vi "index (2).vi"() -> (1 "XY graph visual":cluster{dbl[], dbl[]}(graph))   [LabVIEW 2026]
uses:
  <userlib>/Status.ctl
  <vilib>/Instr/_visa.llb/VISA Flush IO Buffer Mask.ctl
  <vilib>/Instr/_visa.llb/VISA Configure Serial Port (Instr).vi
  <vilib>/Analysis/3filter.llb/Butterworth Filter (DBL).vi
  <vilib>/measure/maspectr.llb/FFT Spectrum (Mag-Phase) for N Chan.vi
  <vilib>/measure/NI_MAPro.lvlib
  <vilib>/Analysis/NI_AALBase.lvlib
panel:
  out "read buffer":string
  out "CRC Error":bool
  out "Spectrum":cluster{"f0":dbl, "df":dbl, "magnitude":dbl[]}[](graph)
  in  "EditCluster":T1={"Horní mezní frekvence"=0.45000000000000007, "Dolní mezní frekvence"=0.0, "filter type"=enum."Lowpass", "applyFilter"=FALSE, "removeFilter"=FALSE, "undoFIlter"=FALSE} {"Horní mezní frekvence" format="%0.2f"}
  out "Waveform Graph Edit":waveform(dbl)[](graph)
  out "Zobrazeni typu signalu":cluster{string, string}
  in  "Exit Button":bool
  out "NewVal":bool
  in  "MereniAZpracovaniSwitch":bool
  in  "Cluster":T2={"Zařízení"="", "Cesta k uloženému souboru"=path "", "Vzorkovací frekvence"=enum."1000", "Record Button"=FALSE, "Stop Button"=FALSE, "A1 signál"=enum."EMG", "A2 signál"=enum."EMG", "A3 signál"=enum."EMG", "A4 signál"=enum."EMG", "A5 signál"=enum."EMG", "A6 signál"=enum."EMG", "Pin s připojeným signálem"=enum."A1"}
  in  "DO 4":bool
  in  "DO 3":bool
  in  "DO 2":bool
  in  "DO 1":bool
  out "tdms file":refnum<k34>
  out "Ylabel and Plot name":cluster{string, string}
  out "Sample Rate Numeric":i32
  out "Consumer":i32
  out "producer":i32
  in  "error in (no error)":errorcluster
  out "Sync Stop":bool=TRUE
  # "Aplikace pro měření a zpracování dat na platformě PLUX BITalino"
  # "Hz"
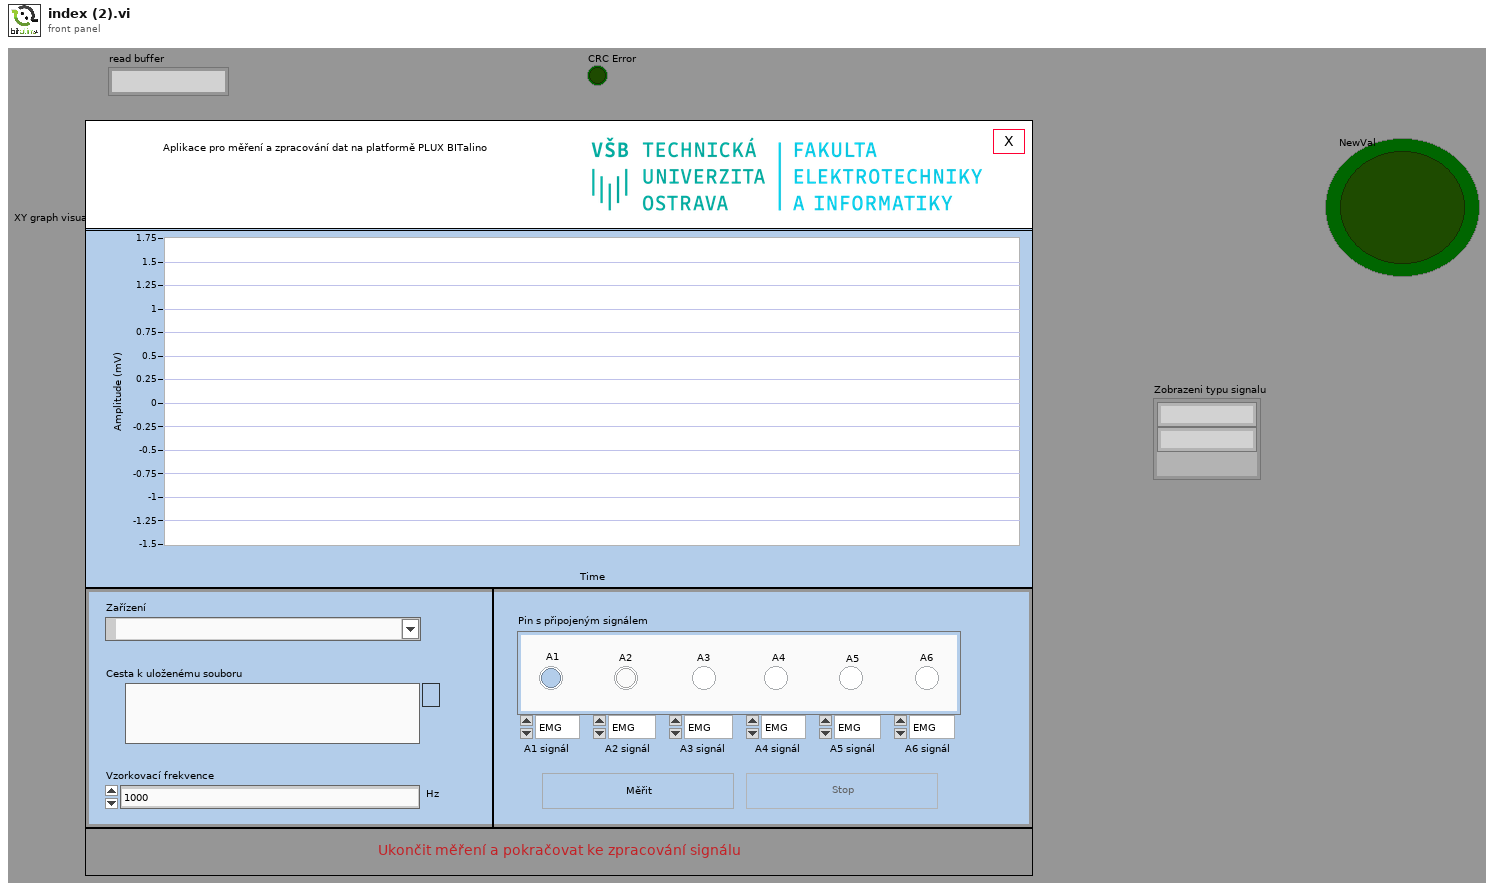
[diagram p1: front panel]
types:
  T1 = cluster{"Horní mezní frekvence":dbl, "Dolní mezní frekvence":dbl, "filter type":enum32{"Lowpass", "Highpass", "Bandpass", "Bandstop"}, "applyFilter":bool, "removeFilter":bool, "undoFIlter":bool}
  T2 = cluster{"Zařízení":refnum<visa-resource-name>, "Cesta k uloženému souboru":path, "Vzorkovací frekvence":enum16{"1", "10", "100", "1000"}, "Record Button":bool, "Stop Button":bool, "A1 signál":enum16{"EMG", "ECG", "EEG", "EDA", "ACC"}, "A2 signál":enum16{"EMG", "ECG", "EEG", "EDA", "ACC"}, "A3 signál":enum16{"EMG", "ECG", "EEG", "EDA", "ACC"}, "A4 signál":enum16{"EMG", "ECG", "EEG", "EDA", "ACC"}, "A5 signál":enum16{"EMG", "ECG", "EEG", "EDA", "ACC"}, "A6 signál":enum16{"EMG", "ECG", "EEG", "EDA", "ACC"}, "Pin s připojeným signálem":enum32{"A1", "A2", "A3", "A4", "A5", "A6"}}
  T3 = enum8{"Enabled", "Disabled", "Disabled and Grayed Out"}
  T4 = enum16{"open", "open or create", "create or replace", "create", "open (read-only)"}
  T5 = typedef "Status.ctl" = enum16{"Initialize", "Edit", "Standby", "Recording", "Exit"}
  T6 = typedef "VISA Flush IO Buffer Mask.ctl" = u16
  T7 = enum32{"Lowpass", "Highpass", "Bandpass", "Bandstop"}
  T8 = cluster{"A1 signál":enum16{"EMG", "ECG", "EEG", "EDA", "ACC"}, "A2 signál":enum16{"EMG", "ECG", "EEG", "EDA", "ACC"}, "A3 signál":enum16{"EMG", "ECG", "EEG", "EDA", "ACC"}, "A4 signál":enum16{"EMG", "ECG", "EEG", "EDA", "ACC"}, "A5 signál":enum16{"EMG", "ECG", "EEG", "EDA", "ACC"}, "A6 signál":enum16{"EMG", "ECG", "EEG", "EDA", "ACC"}}
  T9 = cluster{"Result":dbl, "Result":dbl, "Result":dbl, "Result":dbl, "Result":dbl, "Result":dbl}
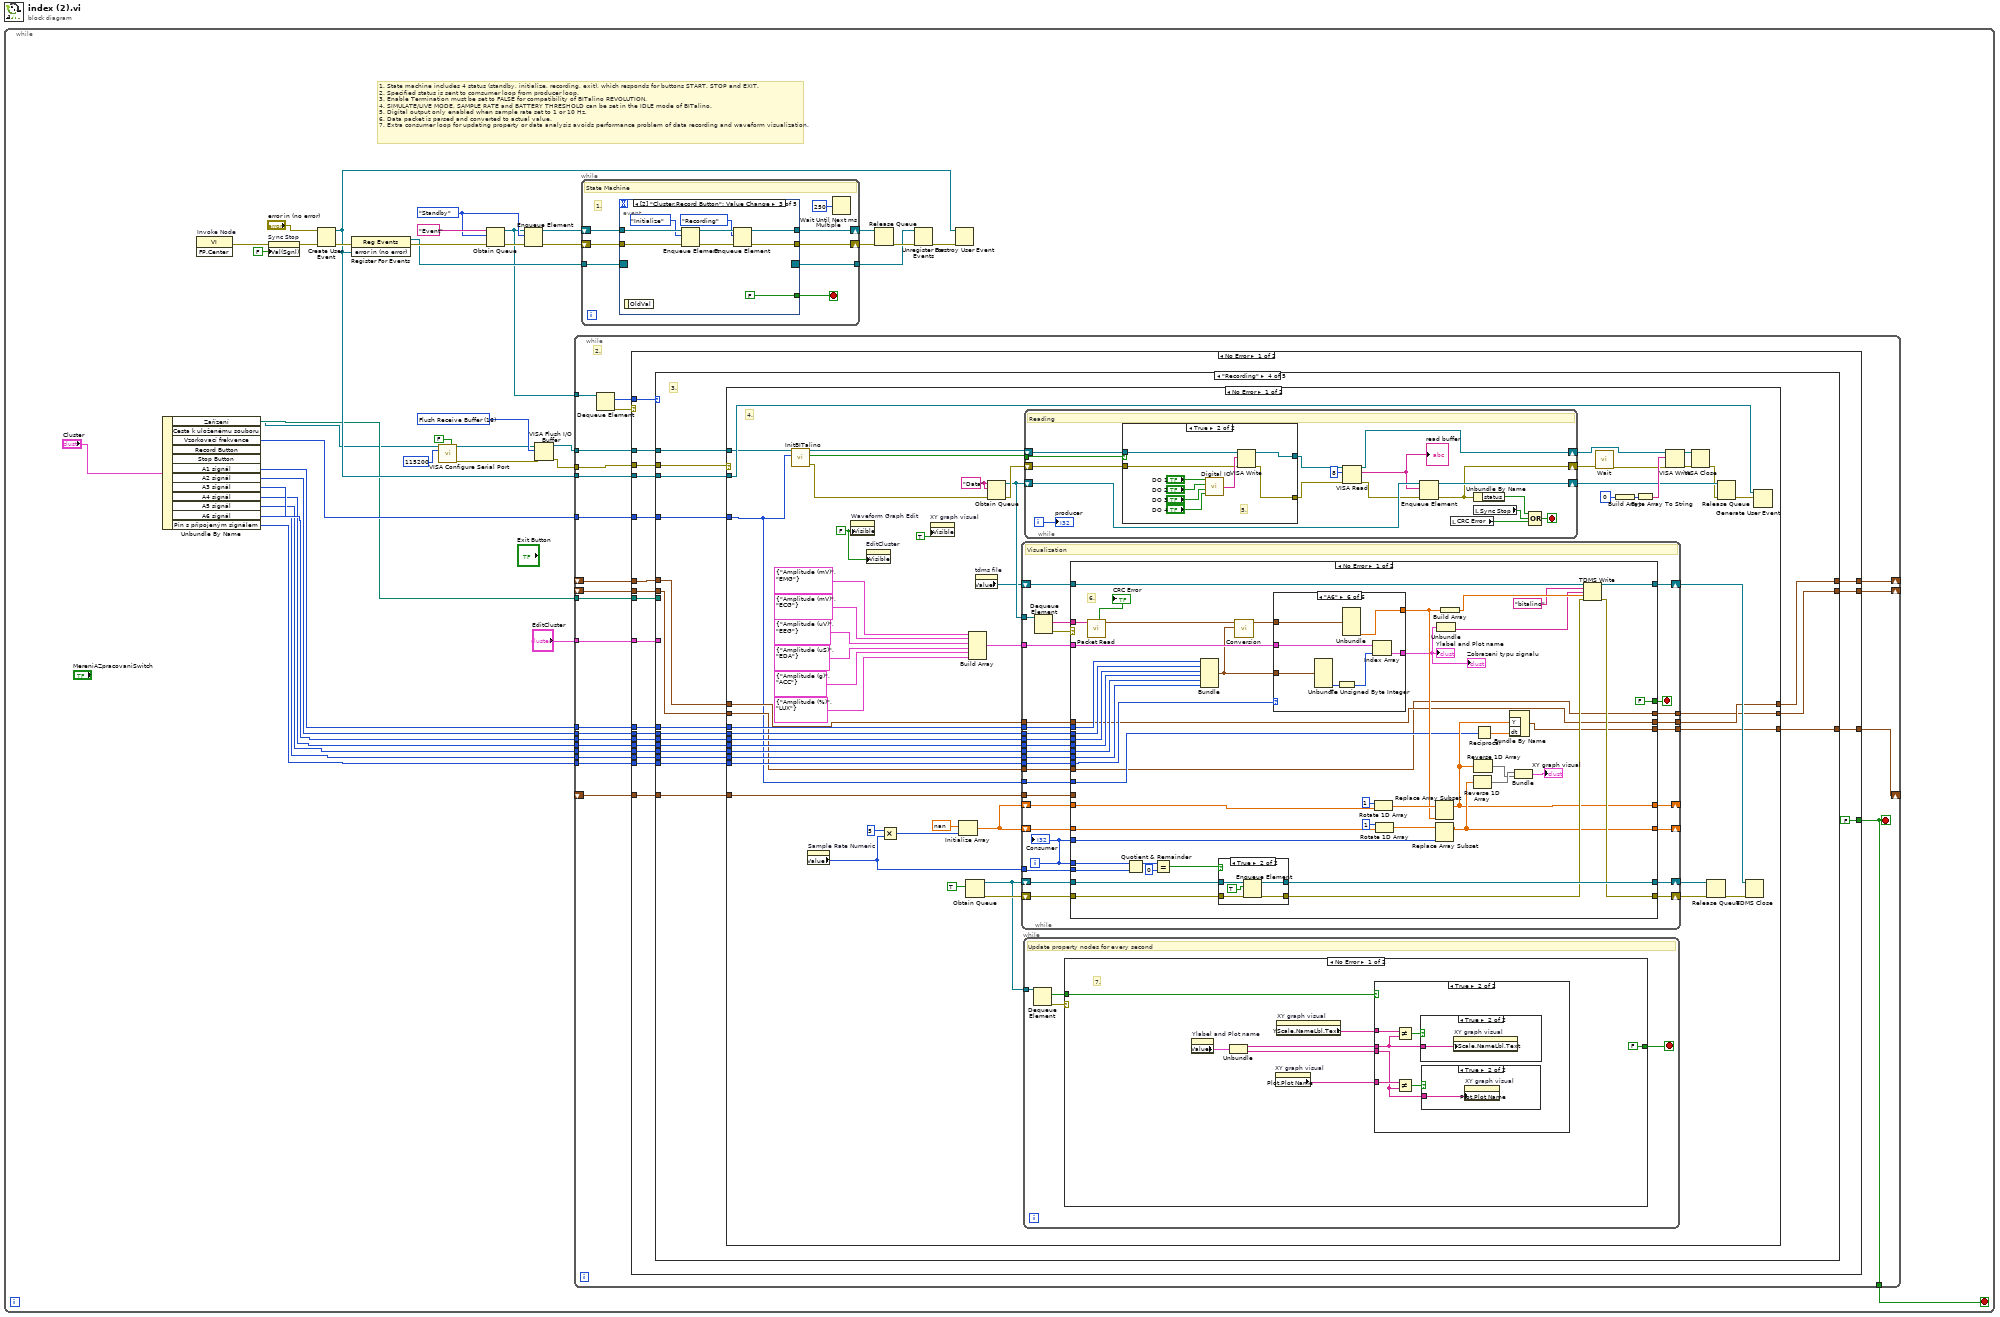
[diagram p0: block diagram]
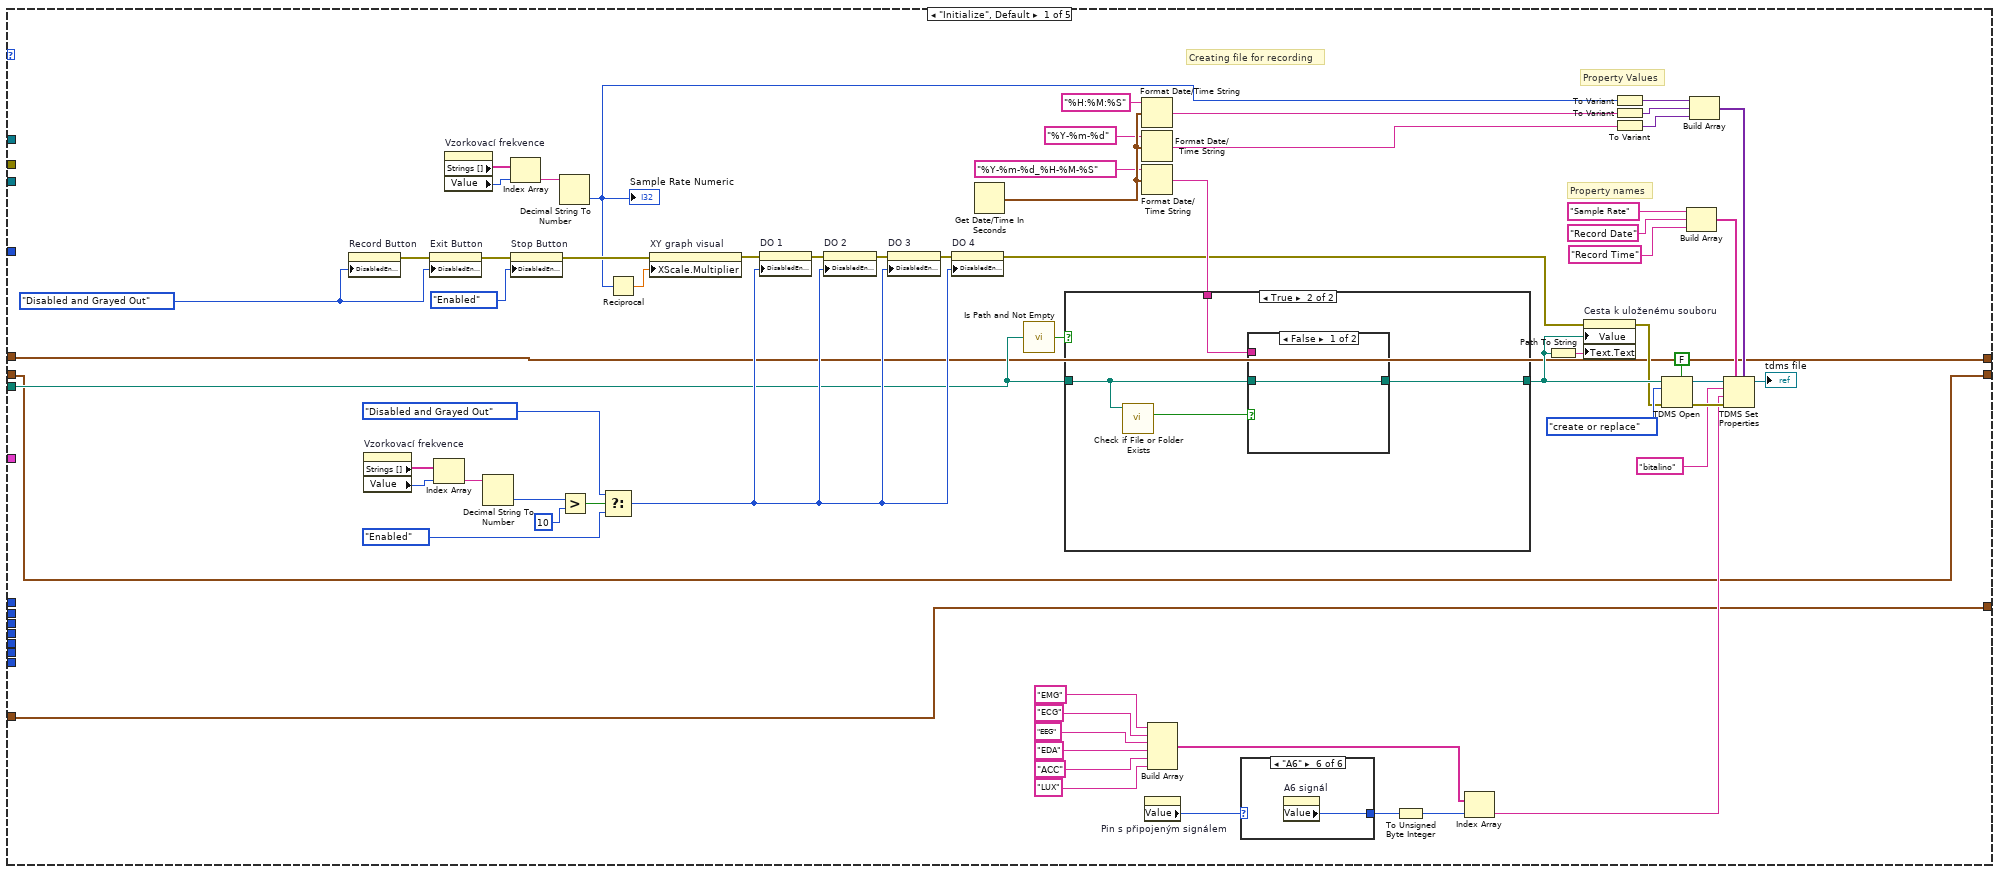
[diagram p2: hidden frame]
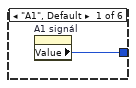
[diagram p3: hidden frame]
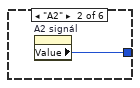
[diagram p4: hidden frame]
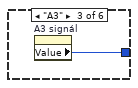
[diagram p5: hidden frame]
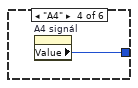
[diagram p6: hidden frame]
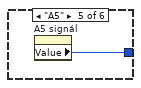
[diagram p7: hidden frame]
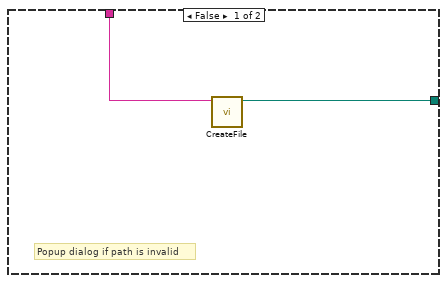
[diagram p8: hidden frame]
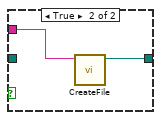
[diagram p9: hidden frame]
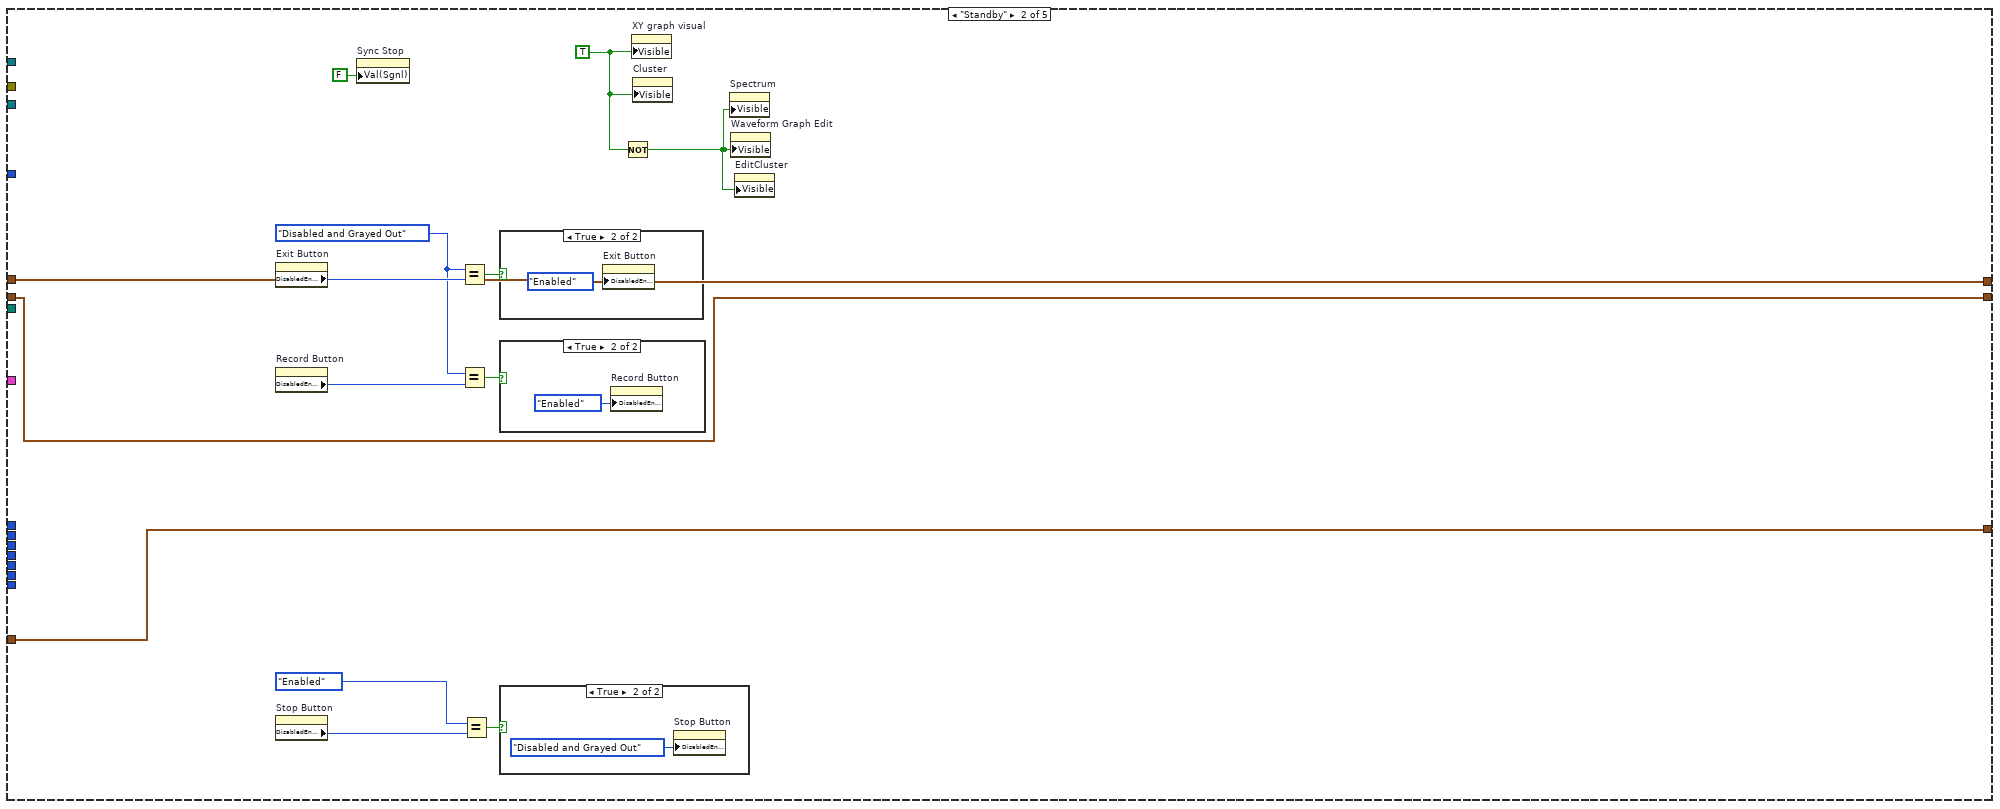
[diagram p10: hidden frame]
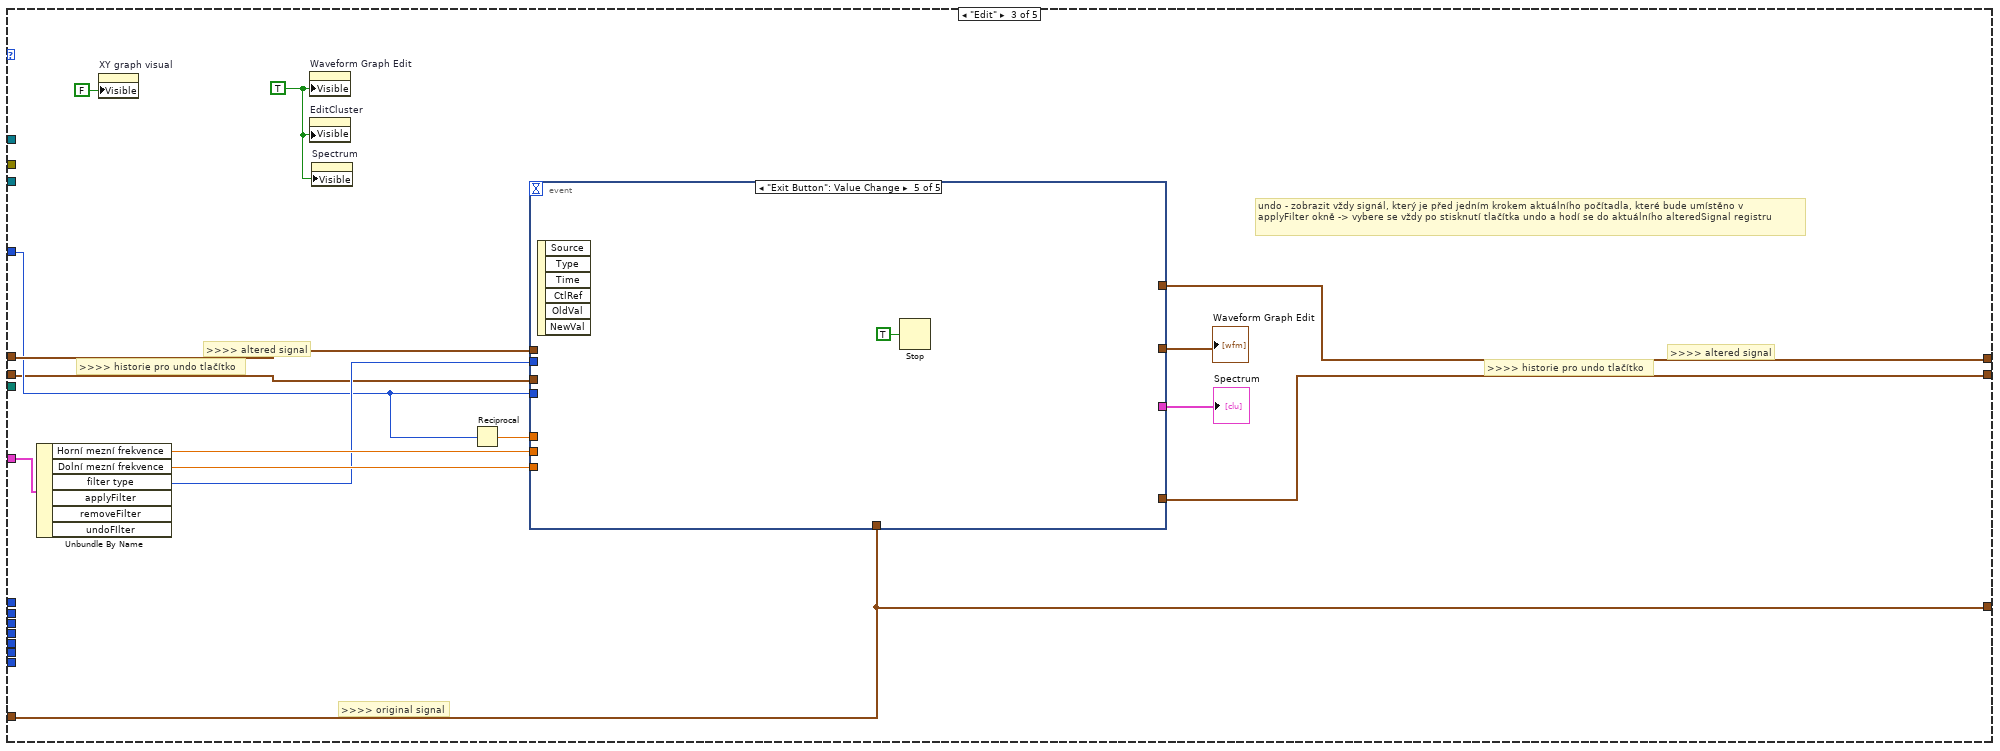
[diagram p14: hidden frame]
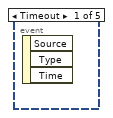
[diagram p15: hidden frame]
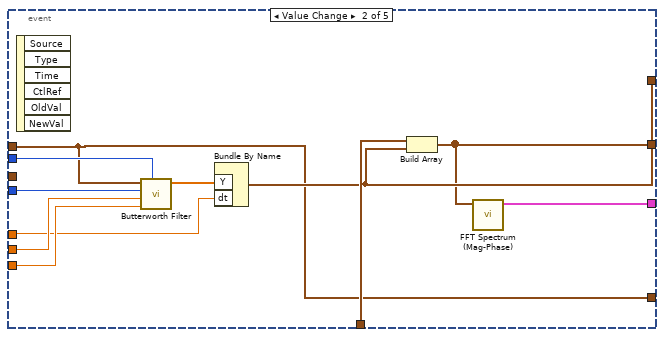
[diagram p16: hidden frame]
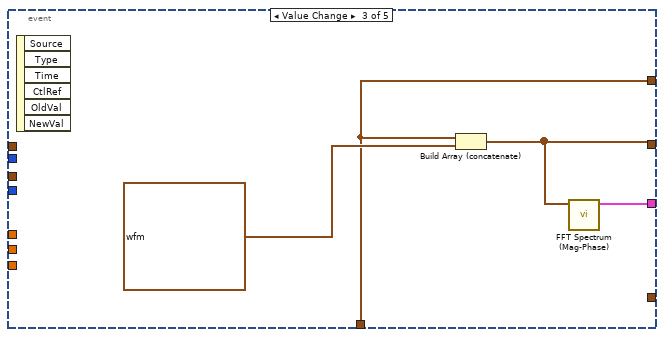
[diagram p17: hidden frame]
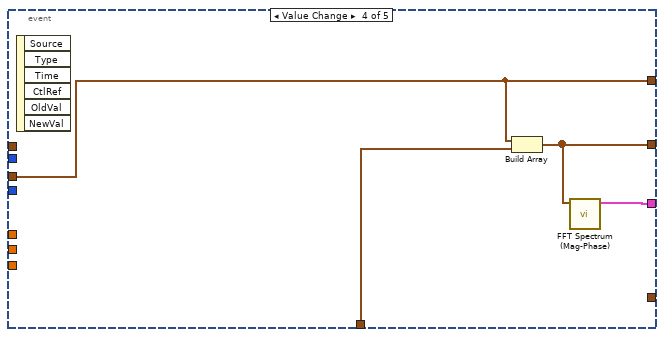
[diagram p18: hidden frame]
diagram:
  n1 = while {
    stop <- w11 stop-if-true
    w4 = T6 16 items=["Flush Receive Buffer"=16, "Write Transmit Buffer to Device"=32, "Flush Receive Buffer (No I/O)"=64, "Flush Transmit Buffer"=128] ("Mask")
    w38 = Status."Standby" ("Enum")
    # "1. State machine includes 4 status (standby, initialize, recording, exit), which responds for buttons START, STOP and EXIT.\n2. Specified status is sent to comsumer loop from producer loop.\n3. Enable Termination must be set to FALSE for compatibility of BITalino REVOLUTION.\n4. SIMULATE/LIVE MODE, SAMPLE RATE and BATTERY THRESHOLD can be set in the IDLE mode of BITalino.\n5. Digital output only enabled when sample rate set to 1 or 10 Hz.\n6. Data packet is parsed and converted to actual value.\n7. Extra consumer loop for updating property or data analysis avoids performance problem of data recording and waveform visualization."
    n2 = Unbundle By Name("Cluster") -> ("Zařízení"=w8:refnum<visa-resource-name>, "Cesta k uloženému souboru"=w12:path, "Vzorkovací frekvence"=w20:enum16{"1", "10", "100", "1000"}, "A1 signál"=w19:enum16{"EMG", "ECG", "EEG", "EDA", "ACC"}, "A2 signál"=w18:enum16{"EMG", "ECG", "EEG", "EDA", "ACC"}, "A3 signál"=w17:enum16{"EMG", "ECG", "EEG", "EDA", "ACC"}, "A4 signál"=w16:enum16{"EMG", "ECG", "EEG", "EDA", "ACC"}, "A5 signál"=w15:enum16{"EMG", "ECG", "EEG", "EDA", "ACC"}, "A6 signál"=w14:enum16{"EMG", "ECG", "EEG", "EDA", "ACC"}, "Pin s připojeným signálem"=w13:enum32{"A1", "A2", "A3", "A4", "A5", "A6"})  [unwired: 2 out]
    n3 = invoke on="Invoke Node" class="VI" method="FP.Center"() -> (error out=w22:errorcluster)  [unwired: 3 in, 2 out]
    n4 = property on="Sync Stop" class="Bool (strict)"(error in=w22, "Val(Sgnl)"=FALSE ("Value (Signaling)")) -> (error out=w31:errorcluster)  [unwired: 1 in, 1 out]
    n5 = Create User Event(user event datatype="error in (no error)", error in=w31) -> (user event=w23:refnum<user-event>, error out=w30:errorcluster)
    n6 = register-events(error in=w30, w23) -> (reference out=w28:refnum<event-registration>, error out=w29:errorcluster)  [unwired: 1 in]
    n7 = call-poly "VISA Configure Serial Port"("VISA resource name"=w8, "Enable Termination\nChar (T)"=FALSE ("Enable Termination\nChar (T)"), "baud rate (9600)"=u32 115200) -> ("VISA resource name out"=w3:refnum<visa-resource-name>, "error out"=w5:errorcluster)  [unwired: 11 in]
    n8 = Obtain Queue(name (unnamed)="Event", element data type=w38, error in (no error)=w29) -> (queue out=w21:refnum<queue>, error out=w34:errorcluster)  [unwired: 2 in, 1 out]
    n9 = Enqueue Element(queue=w21, element=w38, error in (no error)=w34) -> (queue out=w32:refnum<queue>, error out=w33:errorcluster)  [unwired: 1 in, 1 out]
    n10 = VISA Flush I/O Buffer(VISA resource name=w3, mask (16)=w4, error in (no error)=w5) -> (VISA resource name out=w1:refnum<visa-resource-name>, error out=w2:errorcluster)
    n11 = while {
      tunnel: w21 -> [w62]
      tunnel: w23 -> [w42]
      tunnel: w20 -> [w59]
      tunnel: [w58] -> w11
      tunnel: w19 -> [w57]
      tunnel: w18 -> [w56]
      tunnel: w17 -> [w55]
      tunnel: w16 -> [w54]
      tunnel: w15 -> [w53]
      tunnel: w14 -> [w52]
      tunnel: w13 -> [w51]
      tunnel: w12 -> [w50]
      shift-right: [w49] -> _
      shift-left: _ -> [w48]
      tunnel: "EditCluster" -> [w47]
      shift-right: [w46] -> _
      shift-left: _ -> [w45]
      shift-right: [w44] -> _
      shift-left: _ -> [w43]
      tunnel: w2 -> [w41]
      tunnel: w1 -> [w40]
      stop <- w58 stop-if-true
      # "2."
      n12 = Dequeue Element(queue=w62) -> (element=w61:T5, error out=w60:errorcluster)  [unwired: 2 in, 2 out]
      n13 = case shown="No Error" w60 {
        tunnel: w61 -> [w81 _]
        tunnel: [FALSE TRUE] -> w58
        tunnel: w59 -> [w82 _]
        tunnel: w57 -> [w80 _]
        tunnel: w56 -> [w79 _]
        tunnel: w55 -> [w78 _]
        tunnel: w54 -> [w77 _]
        tunnel: w53 -> [w76 _]
        tunnel: w52 -> [w75 _]
        tunnel: w51 -> [w74 _]
        tunnel: w50 -> [w73 _]
        tunnel: [w72 w484] -> w49
        tunnel: w48 -> [w71 w484]
        tunnel: w47 -> [w70 _]
        tunnel: [w69 w483] -> w46
        tunnel: w45 -> [w68 w483]
        tunnel: [w67 w482] -> w44
        tunnel: w43 -> [w66 w482]
        tunnel: w42 -> [w65 _]
        tunnel: w41 -> [w64 _]
        tunnel: w40 -> [w63 _]
        frame No Error {
          n14 = case shown="\"Recording\"" w81 {
            tunnel: w82 -> [_ _ w186 w231 _]
            tunnel: w80 -> [_ _ _ w230 _]
            tunnel: w79 -> [_ _ _ w229 _]
            tunnel: w78 -> [_ _ _ w228 _]
            tunnel: w77 -> [_ _ _ w227 _]
            tunnel: w76 -> [_ _ _ w226 _]
            tunnel: w75 -> [_ _ _ w225 _]
            tunnel: w74 -> [_ _ _ w224 _]
            tunnel: w73 -> [w87 _ _ _ _]
            tunnel: [w86 w167 w183 w223 w479] -> w72
            tunnel: w71 -> [w86 w167 w183 w222 w479]
            tunnel: w70 -> [_ _ w193 _ _]
            tunnel: [w85 w166 w182 w221 w478] -> w69
            tunnel: w68 -> [w85 w166 w191 w220 w478]
            tunnel: [w84 w163 w181 w219 w477] -> w67
            tunnel: w66 -> [w84 w163 w180 w218 w477]
            tunnel: w65 -> [_ _ _ w217 _]
            tunnel: w64 -> [_ _ _ w216 _]
            tunnel: w63 -> [_ _ _ w215 _]
            frame "Initialize", Default {
              w115 = T3."Disabled and Grayed Out" ("Disabled")
              # "Creating file for recording"
              # "Property Values"
              # "Property names"
              n15 = property on="Record Button" class="Bool"("DisabledEnum"=w115) -> (error out=w147:errorcluster)  [unwired: 2 in, 1 out]
              n16 = property on="Vzorkovací frekvence" class="Enum (strict)"() -> ("Strings []"=w105:string[], "Value"=w104:enum16{"1", "10", "100", "1000"})  [unwired: 2 in, 2 out]
              n17 = property on="Exit Button" class="Bool"(error in=w147, "DisabledEnum"=w115) -> (error out=w145:errorcluster)  [unwired: 1 in, 1 out]
              n18 = Index Array "Index Array"(array=w105, index=w104) -> (element=w103:string)
              n19 = property on="Vzorkovací frekvence" class="Enum (strict)"() -> ("Strings []"=w144:string[], "Value"=w143:enum16{"1", "10", "100", "1000"})  [unwired: 2 in, 2 out]
              n20 = Decimal String To Number(string=w103) -> (number=w102:i32)  [unwired: 2 in, 1 out]
              n21 = Index Array(array=w144, index=w143) -> (element=w142:string)
              n22 = property on="Stop Button" class="Bool"(error in=w145, "DisabledEnum"=T3."Enabled" ("Disabled")) -> (error out=w141:errorcluster)  [unwired: 1 in, 1 out]
              n23 = Decimal String To Number(string=w142) -> (number=w114:i32)  [unwired: 2 in, 1 out]
              "Sample Rate Numeric" <- w114
              n24 = Greater?(x=w102, y=10) -> (0:w110:bool)
              n25 = Select(t=T3."Disabled and Grayed Out" ("Disabled"), s=w110, f=T3."Enabled" ("Disabled")) -> (s? t:f=w113:T3)
              n26 = Reciprocal(x=w114) -> (1/x=w140:dbl)
              n27 = property on="XY graph visual" class="XYGraph (strict)"(error in=w141, "XScale.Multiplier"=w140) -> (error out=w101:errorcluster)  [unwired: 1 in, 1 out]
              n28 = property on="DO 1" class="Bool (strict)"(error in=w101, "DisabledEnum"=w113) -> (error out=w108:errorcluster)  [unwired: 1 in, 1 out]
              n29 = property on="DO 2" class="Bool (strict)"(error in=w108, "DisabledEnum"=w113) -> (error out=w107:errorcluster)  [unwired: 1 in, 1 out]
              n30 = property on="DO 3" class="Bool (strict)"(error in=w107, "DisabledEnum"=w113) -> (error out=w106:errorcluster)  [unwired: 1 in, 1 out]
              n31 = property on="DO 4" class="Bool (strict)"(error in=w106, "DisabledEnum"=w113) -> (error out=w100:errorcluster)  [unwired: 1 in, 1 out]
              n32 = Get Date/Time In Seconds() -> (seconds since 1Jan1904=w130:timestamp)
              n33 = call <vilib>:"Is Path and Not Empty.vi"("path"=w87) -> ("Is Path and Not Empty?"=w122:bool)  [unwired: 4 in]
              n34 = Format Date/Time String(time format string (%c)="%H:%M:%S", seconds (now)=w130) -> (date/time string=w135:string)  [unwired: 1 in]
              n35 = Format Date/Time String(time format string (%c)="%Y-%m-%d", seconds (now)=w130) -> (date/time string=w136:string)  [unwired: 1 in]
              n36 = Format Date/Time String(time format string (%c)="%Y-%m-%d_%H-%M-%S", seconds (now)=w130) -> (date/time string=w126:string)  [unwired: 1 in]
              n37 = case shown="True" w122 {
                tunnel: [w154 w157] -> w119
                tunnel: w87 -> [_ w156]
                tunnel: w126 -> [w155 w158]
                frame False {
                  # "Popup dialog if path is invalid"
                  n38 = call "CreateFile.vi"("date/time string"=w155) -> ("appended path"=w154:path)  [unwired: 10 in]
                }
                frame True {
                  n39 = call <vilib>:"Check if File or Folder Exists.vi"("path"=w156) -> ("file or folder exists?"=w159:bool)  [unwired: 8 in, 2 out]
                  n40 = case shown="False" w159 {
                    tunnel: w158 -> [_ w162]
                    tunnel: [w160 w161] -> w157
                    tunnel: w156 -> [w160 _]
                    frame False {
                    }
                    frame True {
                      n41 = call "CreateFile.vi"("date/time string"=w162) -> ("appended path"=w161:path)  [unwired: 10 in]
                    }
                  }
                }
              }
              n42 = property on="Pin s připojeným signálem" class="RadioBtnsControl (strict)"() -> ("Value"=w98:enum32{"A1", "A2", "A3", "A4", "A5", "A6"})  [unwired: 2 in, 2 out]
              n43 = Build Array("EMG", "ECG", "EEG", "EDA", "ACC", "LUX") -> (w89:string[])
              n44 = case shown="\"A6\"" w98 {
                tunnel: [w148 w149 w150 w151 w152 w153] -> w91
                frame "A1", Default {
                  n45 = property on="A1 signál" class="Enum (strict)"() -> ("Value"=w148:enum16{"EMG", "ECG", "EEG", "EDA", "ACC"})  [unwired: 2 in, 2 out]
                }
                frame "A2" {
                  n46 = property on="A2 signál" class="Enum (strict)"() -> ("Value"=w149:enum16{"EMG", "ECG", "EEG", "EDA", "ACC"})  [unwired: 2 in, 2 out]
                }
                frame "A3" {
                  n47 = property on="A3 signál" class="Enum (strict)"() -> ("Value"=w150:enum16{"EMG", "ECG", "EEG", "EDA", "ACC"})  [unwired: 2 in, 2 out]
                }
                frame "A4" {
                  n48 = property on="A4 signál" class="Enum (strict)"() -> ("Value"=w151:enum16{"EMG", "ECG", "EEG", "EDA", "ACC"})  [unwired: 2 in, 2 out]
                }
                frame "A5" {
                  n49 = property on="A5 signál" class="Enum (strict)"() -> ("Value"=w152:enum16{"EMG", "ECG", "EEG", "EDA", "ACC"})  [unwired: 2 in, 2 out]
                }
                frame "A6" {
                  n50 = property on="A6 signál" class="Enum (strict)"() -> ("Value"=w153:enum16{"EMG", "ECG", "EEG", "EDA", "ACC"})  [unwired: 2 in, 2 out]
                }
              }
              n51 = To Unsigned Byte Integer(number=w91) -> (unsigned 8bit integer=w90:u8)
              n52 = Index Array(array=w89, index=w90) -> (element=w88:string)
              n53 = Path To String(path=w119) -> (string=w120:string)
              n54 = property on="Cesta k uloženému souboru" class="Path"(error in=w100, "Value"=w119, "Text.Text"=w120) -> (error out=w118:errorcluster)  [unwired: 1 in, 1 out]
              n55 = To Variant(anything=w114) -> (Variant=w134:variant)
              n56 = To Variant(anything=w135) -> (Variant=w137:variant)
              n57 = To Variant(anything=w136) -> (Variant=w138:variant)
              n58 = TDMS Open(5:FALSE ("create index file? (T)"), 8:w118, 10:T4."create or replace" ("operation (0:open)"), 11:w119) -> (0:w125:errorcluster, 3:w124:refnum<k34>)  [unwired: 3 in]
              n59 = Build Array("Sample Rate", "Record Date", "Record Time") -> (w133:string[])
              n60 = Build Array(w134, w137, w138) -> (w139:variant[])
              n61 = TDMS Set Properties(5:w139, 7:w133, 8:w125, 9:w88, 10:"bitalino", 11:w124) -> (3:→"tdms file":refnum<k34>)  [unwired: 3 out]
            }
            frame "Standby" {
              w165 = TRUE ("Visible")
              w168 = T3."Disabled and Grayed Out" ("Disabled")
              n62 = property on="Exit Button" class="Bool"() -> ("DisabledEnum"=w175:T3)  [unwired: 2 in, 2 out]
              n63 = property on="Record Button" class="Bool"() -> ("DisabledEnum"=w173:T3)  [unwired: 2 in, 2 out]
              n64 = property on="Stop Button" class="Bool"() -> ("DisabledEnum"=w170:T3)  [unwired: 2 in, 2 out]
              n65 = property on="Sync Stop" class="Bool (strict)"("Val(Sgnl)"=FALSE ("Value (Signaling)")) -> ()  [unwired: 2 in, 2 out]
              n66 = Equal?(x=w168, y=w175) -> (x = y?=w174:bool)
              n67 = Equal?(x=w168, y=w173) -> (x = y?=w172:bool)
              n68 = Equal?(x=T3."Enabled" ("Disabled"), y=w170) -> (x = y?=w169:bool)
              n69 = case shown="True" w174 {
                frame False {
                }
                frame True {
                  n70 = property on="Exit Button" class="Bool"("DisabledEnum"=T3."Enabled" ("Disabled")) -> ()  [unwired: 2 in, 2 out]
                }
              }
              n71 = case shown="True" w172 {
                frame False {
                }
                frame True {
                  n72 = property on="Record Button" class="Bool"("DisabledEnum"=T3."Enabled" ("Disabled")) -> ()  [unwired: 2 in, 2 out]
                }
              }
              n73 = case shown="True" w169 {
                frame False {
                }
                frame True {
                  n74 = property on="Stop Button" class="Bool"("DisabledEnum"=T3."Disabled and Grayed Out" ("Disabled")) -> ()  [unwired: 2 in, 2 out]
                }
              }
              n75 = Not(x=w165) -> (.not. x?=w164:bool)
              n76 = property on="XY graph visual" class="XYGraph (strict)"("Visible"=w165) -> ()  [unwired: 2 in, 2 out]
              n77 = property on="Cluster" class="Clust"("Visible"=w165) -> ()  [unwired: 2 in, 2 out]
              n78 = property on="Spectrum" class="WFGraph (strict)"("Visible"=w164) -> ()  [unwired: 2 in, 2 out]
              n79 = property on="Waveform Graph Edit" class="WFGraph (strict)"("Visible"=w164) -> ()  [unwired: 2 in, 2 out]
              n80 = property on="EditCluster" class="Clust"("Visible"=w164) -> ()  [unwired: 2 in, 2 out]
            }
            frame "Edit" {
              w192 = TRUE ("Visible")
              # ">>>> altered signal"
              # ">>>> historie pro undo tlačítko"
              # ">>>> historie pro undo tlačítko"
              # "undo - zobrazit vždy signál, který je před jedním krokem aktuálního počítadla, které bude umístěno v \napplyFilter okně -> vybere se vždy po stisknutí tlačítka undo a hodí se do aktuálního alteredSignal registru"
              # ">>>> altered signal"
              # ">>>> original signal"
              n81 = Unbundle By Name(w193) -> ("Horní mezní frekvence"=w189:dbl, "Dolní mezní frekvence"=w188:dbl, "filter type"=w187:T7)  [unwired: 3 out]
              n82 = property on="XY graph visual" class="XYGraph (strict)"("Visible"=FALSE) -> ()  [unwired: 2 in, 2 out]
              n83 = property on="Waveform Graph Edit" class="WFGraph (strict)"("Visible"=w192) -> ()  [unwired: 2 in, 2 out]
              n84 = property on="EditCluster" class="Clust"("Visible"=w192) -> ()  [unwired: 2 in, 2 out]
              n85 = property on="Spectrum" class="WFGraph (strict)"("Visible"=w192) -> ()  [unwired: 2 in, 2 out]
              n86 = Reciprocal(x=w186) -> (1/x=w190:dbl)
              n87 = event shown="[4] \"Exit Button\": Value Change" {
                selector: _ -> [_ _ _ _ _]
                dyn-events: _ -> [_ _ _ _ _]
                timeout: _ -> [_ _ _ _ _]
                tunnel: w183 -> [_ w204 w206 w212 _]
                tunnel: [_ w203 w206 w213 _] -> w182
                tunnel: w191 -> [_ w195 _ _ _]
                tunnel: w190 -> [_ w199 _ _ _]
                tunnel: w189 -> [_ w202 _ _ _]
                tunnel: w188 -> [_ w201 _ _ _]
                tunnel: w187 -> [_ w200 _ _ _]
                tunnel: w186 -> [_ w198 _ _ _]
                tunnel: [_ w197 w207 w210 _] -> w185
                tunnel: [_ w196 w208 w211 _] -> w184
                tunnel: [_ w195 _ _ _] -> w181
                tunnel: w180 -> [_ _ _ w213 _]
                event Timeout {
                  n88 = event-data() -> ()  [unwired: 1 in, 3 out]
                }
                event "EditCluster.applyFilter": Value Change {
                  n89 = event-data() -> ()  [unwired: 1 in, 6 out]
                  n90 = call-poly <vilib>:"Butterworth Filter.vi"("filter type"=w200, "low cutoff freq: fl"=w201, "high cutoff freq: fh"=w202, "sampling freq: fs"=w198, "X"=w195) -> ("Filtered X"=w205:dbl[])  [unwired: 3 in, 1 out]
                  n91 = Bundle By Name("Y"=w205, "dt"=w199) -> (w203:waveform(dbl))  [unwired: 1 in]
                  n92 = Build Array(w204, w203) -> (w197:waveform(dbl)[])
                  n93 = call-poly <vilib>:"FFT Spectrum (Mag-Phase).vi"("time signals"=w197) -> ("magnitudes"=w196:cluster{"f0":dbl, "df":dbl, "magnitude":dbl[]}[])  [unwired: 6 in, 4 out]
                }
                event "EditCluster.removeFilter": Value Change {
                  n94 = event-data() -> ()  [unwired: 1 in, 6 out]
                  n95 = Build Array (concatenate)(w206, waveform(dbl)[] [{"t0"=timestamp(-3600 s since 1904-01-01), "dt"=10000.0, "Y"=[0.0]}] ("array")) -> (w207:waveform(dbl)[])
                  n96 = call-poly <vilib>:"FFT Spectrum (Mag-Phase).vi"("time signals"=w207) -> ("magnitudes"=w208:cluster{"f0":dbl, "df":dbl, "magnitude":dbl[]}[])  [unwired: 6 in, 4 out]
                }
                event "EditCluster.undoFIlter": Value Change {
                  n97 = event-data() -> ()  [unwired: 1 in, 6 out]
                  n98 = Build Array(w213, w212) -> (w210:waveform(dbl)[])
                  n99 = call-poly <vilib>:"FFT Spectrum (Mag-Phase).vi"("time signals"=w210) -> ("magnitudes"=w211:cluster{"f0":dbl, "df":dbl, "magnitude":dbl[]}[])  [unwired: 6 in, 4 out]
                }
                event "Exit Button": Value Change {
                  n100 = event-data() -> ()  [unwired: 1 in, 6 out]
                  n101 = Stop(stop? (T)=TRUE) -> ()
                }
              }
              "Waveform Graph Edit" <- w185
              "Spectrum" <- w184
            }
            frame "Recording" {
              # "3."
              n102 = case shown="No Error" w216 {
                selector: w216 -> [_ w475]
                tunnel: w217 -> [w273 w476]
                tunnel: w231 -> [w233 _]
                tunnel: w230 -> [w252 _]
                tunnel: w229 -> [w251 _]
                tunnel: w228 -> [w250 _]
                tunnel: w227 -> [w249 _]
                tunnel: w226 -> [w248 _]
                tunnel: w225 -> [w247 _]
                tunnel: w224 -> [w246 _]
                tunnel: [w244 w474] -> w223
                tunnel: w222 -> [w242 w474]
                tunnel: [w241 w473] -> w221
                tunnel: w220 -> [w240 w473]
                tunnel: [w238 w472] -> w219
                tunnel: w218 -> [w237 w472]
                tunnel: w215 -> [w236 _]
                frame No Error {
                  w239 = FALSE ("Visible")
                  w281 = "Data"
                  # "4."
                  n103 = call "InitBITalino.vi"("Sample Rate"=w233, "BITalino"=w236) -> ("error out"=w232:errorcluster, "Digital Output"=w234:bool, "VISA out"=w235:refnum<visa-resource-name>)  [unwired: 7 in]
                  n104 = property on="Sample Rate Numeric" class="DigNum (strict)"() -> ("Value"=w266:i32)  [unwired: 2 in, 2 out]
                  n105 = property on="Waveform Graph Edit" class="WFGraph (strict)"("Visible"=w239) -> ()  [unwired: 2 in, 2 out]
                  n106 = property on="EditCluster" class="Clust"("Visible"=w239) -> ()  [unwired: 2 in, 2 out]
                  n107 = Multiply(x=5, y=w266) -> (x*y=w264:i32)
                  n108 = property on="XY graph visual" class="XYGraph (strict)"("Visible"=TRUE) -> ()  [unwired: 2 in, 2 out]
                  n109 = Initialize Array(nan ("element"), w264) -> (w263:dbl[])
                  n110 = Obtain Queue(element data type=TRUE) -> (queue out=w269:refnum<queue>, error out=w271:errorcluster)  [unwired: 4 in, 1 out]
                  n111 = Build Array(cluster{string, string} {"Amplitude (mV)", "EMG"}, cluster{string, string} {"Amplitude (mV)", "ECG"}, cluster{string, string} {"Amplitude (uV)", "EEG"}, cluster{string, string} {"Amplitude (uS)", "EDA"}, cluster{string, string} {"Amplitude (g)", "ACC"}, cluster{string, string} {"Amplitude (%)", "LUX"}) -> (w256:cluster{string, string}[])
                  n112 = property on="tdms file" class="Ref (strict)"() -> ("Value"=w255:refnum<k34>)  [unwired: 2 in, 2 out]
                  n113 = Obtain Queue(name (unnamed)=w281, element data type=w281, error in (no error)=w232) -> (queue out=w282:refnum<queue>, error out=w283:errorcluster)  [unwired: 2 in, 1 out]
                  n114 = while {
                    tunnel: w282 -> [w337]
                    shift-right: [w332] -> _
                    shift-left: w263 -> [w333]
                    tunnel: w266 -> [w331]
                    shift-right: [w328] -> w268
                    shift-left: w269 -> [w330]
                    shift-right: [w327] -> w267
                    shift-left: w271 -> [w329]
                    shift-right: [w324] -> _
                    shift-left: w263 -> [w326]
                    tunnel: w256 -> [w323]
                    shift-right: [w321] -> w253
                    shift-left: w255 -> [w322]
                    tunnel: w252 -> [w320]
                    tunnel: w251 -> [w319]
                    tunnel: w250 -> [w318]
                    tunnel: w249 -> [w317]
                    tunnel: w248 -> [w316]
                    tunnel: w247 -> [w315]
                    tunnel: w246 -> [w314]
                    tunnel: w233 -> [w313]
                    tunnel: [w312] -> w244
                    tunnel: w242 -> [w311]
                    tunnel: [w310] -> w241
                    tunnel: w240 -> [w309]
                    tunnel: [w308] -> w238
                    tunnel: w237 -> [w307]
                    i -> [w325]
                    stop <- w335 stop-if-true
                    # "Visualization"
                    n115 = Dequeue Element(queue=w337) -> (element=w334:string, error out=w336:errorcluster)  [unwired: 2 in, 2 out]
                    n116 = case shown="No Error" w336 {
                      tunnel: [FALSE TRUE] -> w335
                      tunnel: w334 -> [w360 _]
                      tunnel: w333 -> [w373 w442]
                      tunnel: [w346 w442] -> w332
                      tunnel: w331 -> [w374 _]
                      tunnel: w325 -> [w379 _]
                      tunnel: w330 -> [w382 w441]
                      tunnel: w329 -> [w381 w440]
                      tunnel: [w380 w441] -> w328
                      tunnel: [w361 w440] -> w327
                      tunnel: w326 -> [w370 w439]
                      tunnel: w325 -> [w369 _]
                      tunnel: [w349 w439] -> w324
                      tunnel: w323 -> [w368 _]
                      tunnel: w322 -> [w366 w438]
                      tunnel: [w365 w438] -> w321
                      tunnel: w320 -> [w356 _]
                      tunnel: w319 -> [w355 _]
                      tunnel: w318 -> [w354 _]
                      tunnel: w317 -> [w353 _]
                      tunnel: w316 -> [w352 _]
                      tunnel: w315 -> [w351 _]
                      tunnel: w314 -> [w350 _]
                      tunnel: w313 -> [w344 _]
                      tunnel: [w343 w437] -> w312
                      tunnel: w311 -> [_ w437]
                      tunnel: [w342 w436] -> w310
                      tunnel: w309 -> [w342 w436]
                      tunnel: [w341 w435] -> w308
                      tunnel: w307 -> [w341 w435]
                      frame No Error {
                        # "6."
                        n117 = call "Packet Read.vi"("Packets"=w360) -> ("Analog Channels"=w359:cluster{u16, u16, u16, u16, u16, u16}, "CRC Error"=→"CRC Error":bool)  [unwired: 7 in, 2 out]
                        n118 = Quotient & Remainder(x=w379, y=w374) -> (x-y*floor(x/y)=w378:i32)  [unwired: 1 out]
                        n119 = Equal?(x=w378, y=0) -> (x = y?=w376:bool)
                        n120 = Bundle "Bundle"("A1 signál"=w356, "A2 signál"=w355, "A3 signál"=w354, "A4 signál"=w353, "A5 signál"=w352, "A6 signál"=w351) -> (w367:T8)  [unwired: 1 in]
                        n121 = case shown="True" w376 {
                          tunnel: w382 -> [w387 w392]
                          tunnel: w381 -> [w386 w391]
                          tunnel: [w387 w390] -> w380
                          tunnel: [w386 w389] -> w364
                          frame False {
                          }
                          frame True {
                            n122 = Enqueue Element(queue=w392, element=TRUE, error in (no error)=w391) -> (queue out=w390:refnum<queue>, error out=w389:errorcluster)  [unwired: 1 in, 1 out]
                          }
                        }
                        n123 = call "Conversion.vi"("Sensor Type"=w367, "Analog Channels"=w359) -> ("Converted Values"=w384:T9)  [unwired: 8 in, 1 out]
                        n124 = case shown="\"A6\"" w350 {
                          tunnel: w384 -> [w399 w406 w413 w420 w427 w434]
                          tunnel: [w398 w405 w412 w419 w426 w433] -> w363
                          tunnel: w368 -> [w394 w401 w408 w416 w422 w430]
                          tunnel: w367 -> [w397 w403 w410 w417 w424 w431]
                          tunnel: [w393 w400 w409 w415 w423 w429] -> w347
                          frame "A1", Default {
                            n125 = Unbundle(w397) -> ("A1 signál"=w395:enum16{"EMG", "ECG", "EEG", "EDA", "ACC"})  [unwired: 5 out]
                            n126 = To Unsigned Byte Integer(number=w395) -> (unsigned 8bit integer=w396:u8)
                            n127 = Unbundle(w399) -> ("Result"=w398:dbl)  [unwired: 5 out]
                            n128 = Index Array(array=w394, index=w396) -> (element=w393:cluster{string, string})
                          }
                          frame "A2" {
                            n129 = Unbundle(w403) -> ("A2 signál"=w402:enum16{"EMG", "ECG", "EEG", "EDA", "ACC"})  [unwired: 5 out]
                            n130 = To Unsigned Byte Integer(number=w402) -> (unsigned 8bit integer=w404:u8)
                            n131 = Unbundle(w406) -> ("Result"=w405:dbl)  [unwired: 5 out]
                            n132 = Index Array(array=w401, index=w404) -> (element=w400:cluster{string, string})
                          }
                          frame "A3" {
                            n133 = Unbundle(w410) -> ("A3 signál"=w407:enum16{"EMG", "ECG", "EEG", "EDA", "ACC"})  [unwired: 5 out]
                            n134 = To Unsigned Byte Integer(number=w407) -> (unsigned 8bit integer=w411:u8)
                            n135 = Unbundle(w413) -> ("Result"=w412:dbl)  [unwired: 5 out]
                            n136 = Index Array(array=w408, index=w411) -> (element=w409:cluster{string, string})
                          }
                          frame "A4" {
                            n137 = Unbundle(w417) -> ("A4 signál"=w414:enum16{"EMG", "ECG", "EEG", "EDA", "ACC"})  [unwired: 5 out]
                            n138 = To Unsigned Byte Integer(number=w414) -> (unsigned 8bit integer=w418:u8)
                            n139 = Unbundle(w420) -> ("Result"=w419:dbl)  [unwired: 5 out]
                            n140 = Index Array(array=w416, index=w418) -> (element=w415:cluster{string, string})
                          }
                          frame "A5" {
                            n141 = Unbundle(w424) -> ("A5 signál"=w421:enum16{"EMG", "ECG", "EEG", "EDA", "ACC"})  [unwired: 5 out]
                            n142 = Unbundle(w427) -> ("Result"=w426:dbl)  [unwired: 5 out]
                            n143 = To Unsigned Byte Integer(number=w421) -> (unsigned 8bit integer=w425:u8)
                            n144 = Index Array(array=w422, index=w425) -> (element=w423:cluster{string, string})
                          }
                          frame "A6" {
                            n145 = Unbundle(w431) -> ("A6 signál"=w428:enum16{"EMG", "ECG", "EEG", "EDA", "ACC"})  [unwired: 5 out]
                            n146 = To Unsigned Byte Integer(number=w428) -> (unsigned 8bit integer=w432:u8)
                            n147 = Unbundle(w434) -> ("Result"=w433:dbl)  [unwired: 5 out]
                            n148 = Index Array(array=w430, index=w432) -> (element=w429:cluster{string, string})
                          }
                        }
                        "Ylabel and Plot name" <- w347
                        "Zobrazeni typu signalu" <- w347
                        n149 = Rotate 1D Array(1:w373, 2:1 ("n")) -> (0:w375:dbl[])
                        n150 = Rotate 1D Array(1:w370, 2:1 ("n")) -> (0:w371:dbl[])
                        n151 = Replace Array Subset(array=w375, new element=w363) -> (w346:dbl[])  [unwired: 1 in]
                        n152 = Replace Array Subset(array=w371, new element=w369) -> (w349:dbl[])  [unwired: 1 in]
                        n153 = Unbundle(w347) -> (w358:string)  [unwired: 1 out]
                        n154 = Build Array(w363) -> (w362:dbl[])
                        n155 = Reverse 1D Array(array=w349) -> (reversed array=w340:dbl[])
                        n156 = Reverse 1D Array(array=w346) -> (reversed array=w339:dbl[])
                        n157 = Reciprocal(x=w344) -> (1/x=w345:dbl)
                        n158 = Bundle By Name("Y"=w346, "dt"=w345) -> (w343:waveform(dbl))  [unwired: 1 in]
                        n159 = Bundle(w340, w339) -> (→"XY graph visual":cluster{dbl[], dbl[]})  [unwired: 1 in]
                        n160 = TDMS Write(0:w366, 5:"bitalino", 7:w358, 9:w362, 11:w364) -> (4:w365:refnum<k34>, 15:w361:errorcluster)  [unwired: 1 in, 2 out]
                      }
                      frame Error {
                      }
                    }
                    "Consumer" <- w325
                  }
                  n161 = while {
                    tunnel: w269 -> [w290]
                    stop <- w287 stop-if-true
                    # "Update property nodes for every second"
                    n162 = Dequeue Element(queue=w290) -> (element=w288:bool, error out=w289:errorcluster)  [unwired: 2 in, 2 out]
                    n163 = case shown="No Error" w289 {
                      tunnel: w288 -> [w294 _]
                      tunnel: [FALSE TRUE] -> w287
                      frame No Error {
                        # "7."
                        n164 = property on="Ylabel and Plot name" class="Clust (strict)"() -> ("Value"=w297:cluster{string, string})  [unwired: 2 in, 2 out]
                        n165 = Unbundle(w297) -> (w296:string, w295:string)
                        n166 = property on="XY graph visual" class="XYGraph (strict)"() -> ("Plot.Plot Name"=w291:string)  [unwired: 2 in, 2 out]
                        n167 = property on="XY graph visual" class="XYGraph (strict)"() -> ("YScale.NameLbl.Text"=w292:string)  [unwired: 2 in, 2 out]
                        n168 = case shown="True" w294 {
                          tunnel: w292 -> [_ w303]
                          tunnel: w291 -> [_ w299]
                          tunnel: w296 -> [_ w300]
                          tunnel: w295 -> [_ w298]
                          frame False {
                          }
                          frame True {
                            n169 = Not Equal?(x=w303, y=w300) -> (x != y?=w301:bool)
                            n170 = Not Equal?(x=w299, y=w298) -> (x != y?=w302:bool)
                            n171 = case shown="True" w301 {
                              tunnel: w300 -> [_ w305]
                              frame False {
                              }
                              frame True {
                                n172 = property on="XY graph visual" class="XYGraph (strict)"("YScale.NameLbl.Text"=w305) -> ()  [unwired: 2 in, 2 out]
                              }
                            }
                            n173 = case shown="True" w302 {
                              tunnel: w298 -> [_ w304]
                              frame False {
                              }
                              frame True {
                                n174 = property on="XY graph visual" class="XYGraph (strict)"("Plot.Plot Name"=w304) -> ()  [unwired: 2 in, 2 out]
                              }
                            }
                          }
                        }
                      }
                      frame Error {
                      }
                    }
                  }
                  n175 = while {
                    shift-right: [w458] -> w277
                    shift-left: w283 -> [w453]
                    shift-right: [w459] -> w280
                    shift-left: w282 -> [w460]
                    shift-right: [w444] -> w279
                    shift-left: w235 -> [w452]
                    tunnel: w234 -> [w451]
                    i -> [w457]
                    stop <- w456 stop-if-true
                    # "Reading"
                    n176 = case shown="True" w451 {
                      tunnel: w453 -> [w462 w466]
                      tunnel: w452 -> [w461 w465]
                      tunnel: [w462 w463] -> w448
                      tunnel: [w461 w464] -> w449
                      frame False {
                      }
                      frame True {
                        # "5."
                        n177 = call "Digital IO.vi"("DO 4"="DO 4", "DO 3"="DO 3", "DO in"="DO 2", "DO 1"="DO 1") -> ("string"=w471:string)
                        n178 = VISA Write(VISA resource name=w465, write buffer=w471, error in (no error)=w466) -> (VISA resource name out=w464:refnum<visa-resource-name>, error out=w463:errorcluster)  [unwired: 1 out]
                      }
                    }
                    n179 = VISA Read(VISA resource name=w449, byte count=u32 8, error in (no error)=w448) -> (VISA resource name out=w444:refnum<visa-resource-name>, read buffer=w446:string, error out=w447:errorcluster)  [unwired: 1 out]
                    "read buffer" <- w446
                    n180 = Enqueue Element(queue=w460, element=w446, error in (no error)=w447) -> (queue out=w459:refnum<queue>, error out=w458:errorcluster)  [unwired: 1 in, 1 out]
                    n181 = local read "CRC Error"() -> (w450:bool)
                    n182 = Unbundle By Name(w458) -> ("status"=w454:bool)
                    n183 = local read "Sync Stop"() -> (w455:bool)
                    n184 = Compound Arithmetic op=OR(w454, w455, w450) -> (w456:bool)
                    "producer" <- w457
                  }
                  n185 = call "Wait.vi"("error in (no error)"=w277) -> ("error out"=w278:errorcluster)  [unwired: 10 in]
                  n186 = Build Array(u8 0) -> (w285:u8[])
                  n187 = Byte Array To String(unsigned byte array=w285) -> (string=w284:string)
                  n188 = VISA Write(VISA resource name=w279, write buffer=w284, error in (no error)=w278) -> (VISA resource name out=w275:refnum<visa-resource-name>, error out=w276:errorcluster)  [unwired: 1 out]
                  n189 = VISA Close(VISA resource name=w275, error in (no error)=w276) -> (error out=w274:errorcluster)
                  n190 = Release Queue(queue=w268, error in (no error)=w267) -> (error out=w254:errorcluster)  [unwired: 1 in, 2 out]
                  n191 = Release Queue(queue=w280, error in (no error)=w274) -> (error out=w272:errorcluster)  [unwired: 1 in, 2 out]
                  n192 = TDMS Close(8:w254, 11:w253) -> ()  [unwired: 2 out]
                  n193 = Generate User Event(user event=w273, event data cluster=w272) -> ()  [unwired: 2 in, 2 out]
                }
                frame Error {
                  n194 = Generate User Event(user event=w476, event data cluster=w475) -> ()  [unwired: 2 in, 2 out]
                }
              }
            }
            frame "Exit" {
              n195 = flat-sequence {
                frame #0 {
                  n196 = property on="Stop Button" class="Bool"("DisabledEnum"=T3."Enabled" ("Disabled")) -> ()  [unwired: 2 in, 2 out]
                }
                frame #1 {
                  n197 = Stop(stop? (T)=TRUE) -> ()
                }
              }
            }
          }
        }
        frame Error {
        }
      }
    }
    n198 = while {
      shift-right: [w490] -> w36
      shift-left: w32 -> [w493]
      shift-right: [w491] -> w35
      shift-left: w33 -> [w492]
      tunnel: w28 -> [w487]
      tunnel: [w486] -> w25
      stop <- w489 stop-if-true
      # "1."
      # "State Machine"
      n199 = event shown="[2] \"Cluster.Record Button\": Value Change" {
        selector: w487 -> [_ _ _ _ _]
        dyn-events: [_ _ _ _ _] -> w486
        timeout: _ -> [_ _ _ _ _]
        tunnel: w493 -> [w500 w504 w516 w521 w526]
        tunnel: w492 -> [w497 w506 w515 w519 w524]
        tunnel: [w494 w507 w510 w518 w523] -> w491
        tunnel: [w501 w505 w512 w520 w525] -> w490
        tunnel: [FALSE TRUE FALSE _ _] -> w489
        event "Cluster.Stop Button": Value Change {
          n200 = event-data() -> ()  [unwired: 1 in, 5 out]
          n201 = Enqueue Element(queue=w500, element=Status."Standby" ("Enum"), error in (no error)=w497) -> (queue out=w501:refnum<queue>, error out=w495:errorcluster)  [unwired: 1 in, 1 out]
          n202 = property on="Sync Stop" class="Bool (strict)"(error in=w495, "Val(Sgnl)"=TRUE) -> (error out=w494:errorcluster)  [unwired: 1 in, 1 out]
        }
        event "Exit Button": Value Change {
          n203 = event-data() -> ()  [unwired: 1 in, 5 out]
          n204 = Enqueue Element(queue=w504, element=Status."Exit" ("Enum"), error in (no error)=w506) -> (queue out=w505:refnum<queue>, error out=w507:errorcluster)  [unwired: 1 in, 1 out]
        }
        event "Cluster.Record Button": Value Change {
          n205 = event-data() -> ()  [unwired: 1 in, 1 out]
          n206 = Enqueue Element(queue=w516, element=Status."Initialize" ("Enum"), error in (no error)=w515) -> (queue out=w513:refnum<queue>, error out=w511:errorcluster)  [unwired: 1 in, 1 out]
          n207 = Enqueue Element(queue=w513, element=Status."Recording" ("Enum"), error in (no error)=w511) -> (queue out=w512:refnum<queue>, error out=w510:errorcluster)  [unwired: 1 in, 1 out]
        }
        event "MereniAZpracovaniSwitch": Value Change {
          n208 = event-data() -> ("OldVal"=w522:bool)  [unwired: 1 in]
          "NewVal" <- w522
          n209 = property on="Cluster" class="Clust"("Visible"=w522) -> ()  [unwired: 2 in, 2 out]
          n210 = Enqueue Element(queue=w521, element=Status."Edit", error in (no error)=w519) -> (queue out=w520:refnum<queue>, error out=w518:errorcluster)  [unwired: 1 in, 1 out]
        }
        event User Event {
          n211 = event-data() -> ()  [unwired: 1 in, 1 out]
          n212 = Enqueue Element(queue=w526, element=Status."Standby" ("Enum"), error in (no error)=w524) -> (queue out=w525:refnum<queue>, error out=w523:errorcluster)  [unwired: 1 in, 1 out]
        }
      }
      n213 = Wait Until Next ms Multiple(millisecond multiple=u32 250) -> ()  [unwired: 1 out]
    }
    n214 = Release Queue(queue=w36, error in (no error)=w35) -> (error out=w26:errorcluster)  [unwired: 1 in, 2 out]
    n215 = Unregister For Events(event registration refnum=w25, error in=w26) -> (error out=w24:errorcluster)
    n216 = Destroy User Event(user event=w23, error in=w24) -> ()  [unwired: 1 out]
  }
